vi "Worker List UI.vi"(11 "Opened from Block":bool) -> (3 "Selected Worker Lib":path)   [LabVIEW 2022 SP3, in "FlexBlocks Support.lvlib"]
uses:
  FlexBlocks Support.lvlib
  <vilib>/IlluminatedG/IG AutoComplete/AutoComplete/AutoComplete.lvlib
panel:
  out "Prompt":string
  in  "Select Worker":bool
  in  "Refresh Workers":bool
  in  "Refresh Worker":bool
  out "Icon":picture
  in  "New Variant":bool
  in  "Enable Variants":bool
  in  "Open Worker":bool
  in  "Values":string(tree)
  in  "New Worker":bool
  in  "Variant":i32(listbox)
  in  "Worker Search":string
  in  "Clear Search":bool
  out "Worker Name":string
  in  "Workers":i32(listbox)
  # "No variants for the selected worker"
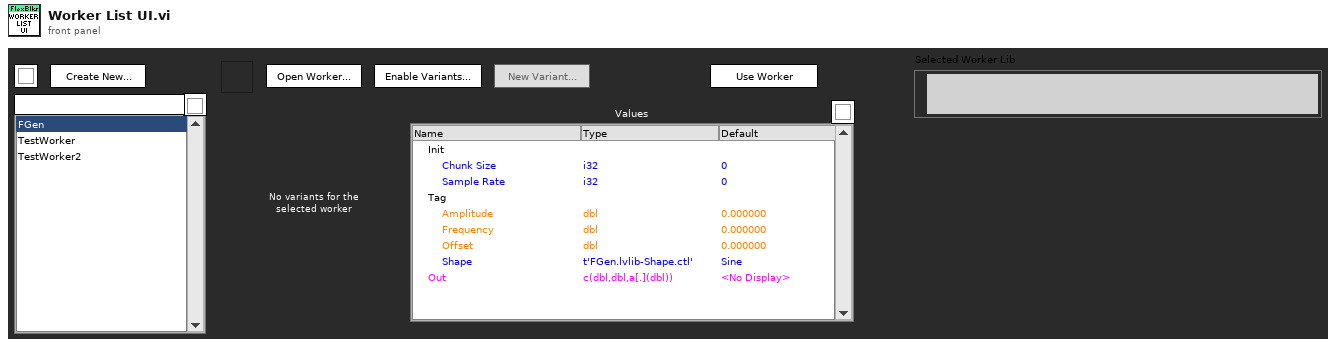
[diagram p1: front panel]
types:
  T1 = typedef "FlexBlocks Support.lvlib/UI State.ctl" = enum16{"Init", "Load", "Ready", "Run", "Cleanup", "Close"}
  T2 = enum8{"Enabled", "Disabled", "Disabled and Grayed Out"}
  T3 = enum32{"Invalid", "Standard", "Closed", "Hidden", "Minimized", "Maximized"}
  T4 = typedef "FlexBlocks Support.lvlib/Action Selections.ctl" = cluster{"Init":bool, "Start":bool, "Run":bool, "Stop":bool, "Close":bool}
  T5 = typedef "FlexBlocks Support.lvlib/Worker Info.ctl" = cluster{"Name":string, "Icon":T6, "Index":i32, "Variants":map{string, T7}}
  T6 = typedef "imagedata.ctl" = cluster{"image type":i32, "image depth":i32, "image":u8[], "mask":u8[], "colors":u32[], "Rectangle":cluster{"left":i16, "top":i16, "right":i16, "bottom":i16}}
  T7 = typedef "FlexBlocks Support.lvlib/Worker Variant.ctl" = cluster{"Name":string, "Icon":T6}
  T8 = typedef "FlexBlocks Support.lvlib/Type Descriptor.ctl" = cluster{"Name":string, "Direction":T9, "Default":variant, "Min":variant, "Max":variant, "Step":variant, "Value Mode":T10, "Color":u32, "Options":string[], "Type String":string, "Item Path":path, "Required":bool, "Connpane Index":i32, "Special Terminal":T11, "Sort":i32}
  T9 = typedef "FlexBlocks Support.lvlib/Terminal Direction.ctl" = enum16{"Sink", "Source"}
  T10 = typedef "FlexBlocks Support.lvlib/Value Mode.ctl" = enum16{"Normal", "Range", "Select"}
  T11 = typedef "FlexBlocks Support.lvlib/Special Terminal.ctl" = enum16{"None", "Action", "Init", "Tag", "State in", "State out", "Error"}
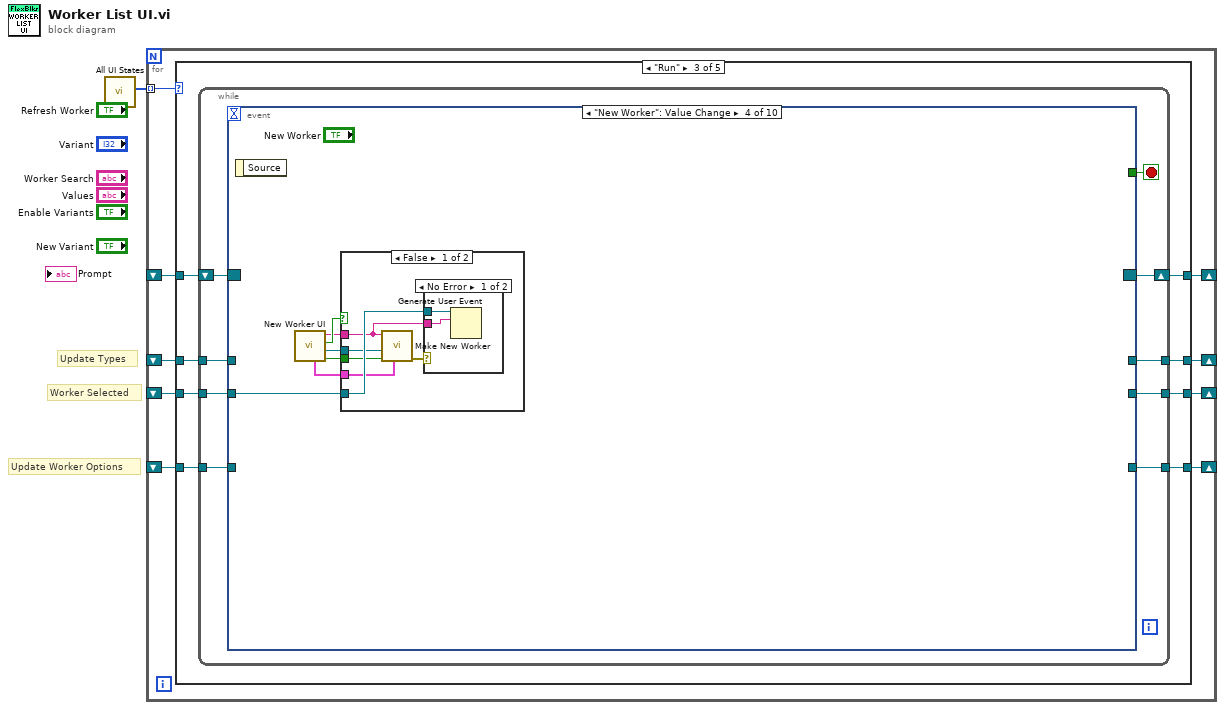
[diagram p0: block diagram]
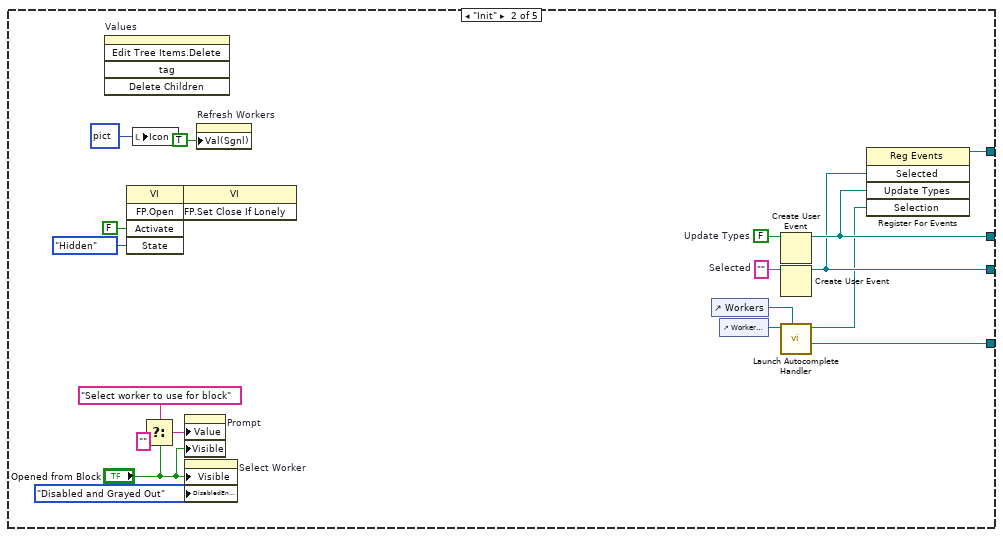
[diagram p3: hidden frame]
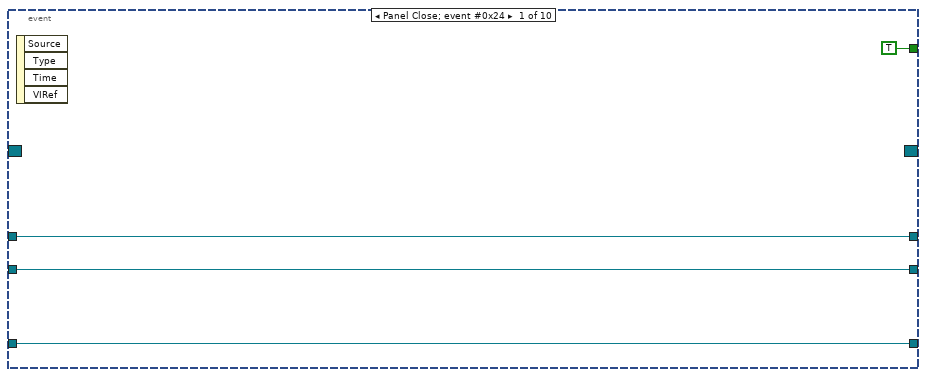
[diagram p4: hidden frame]
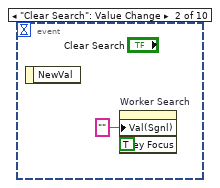
[diagram p5: hidden frame]
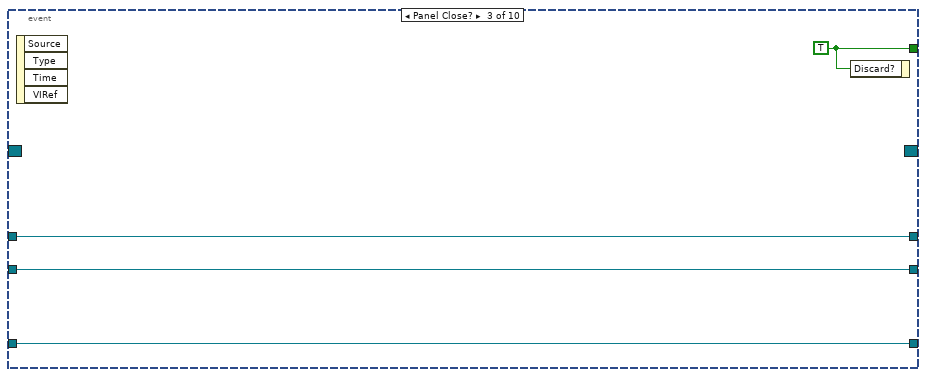
[diagram p6: hidden frame]
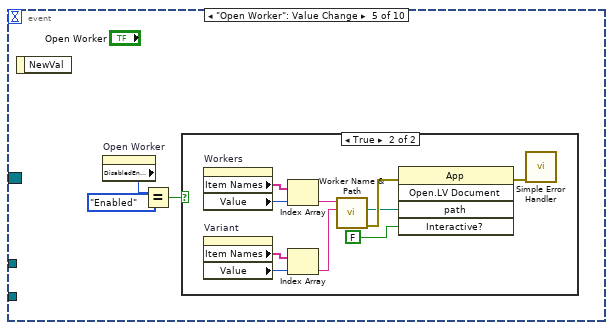
[diagram p9: hidden frame]
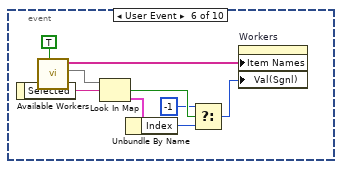
[diagram p11: hidden frame]
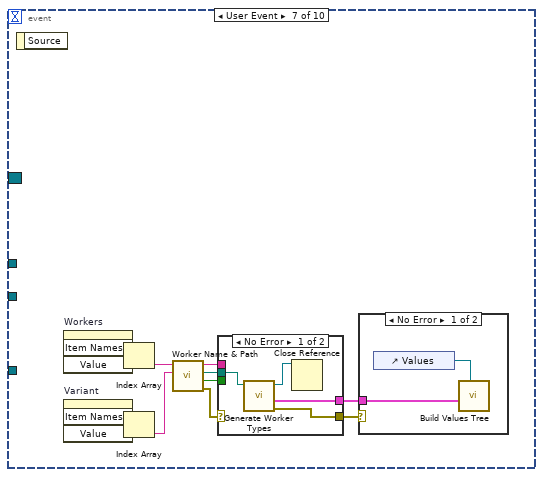
[diagram p12: hidden frame]
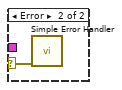
[diagram p13: hidden frame]
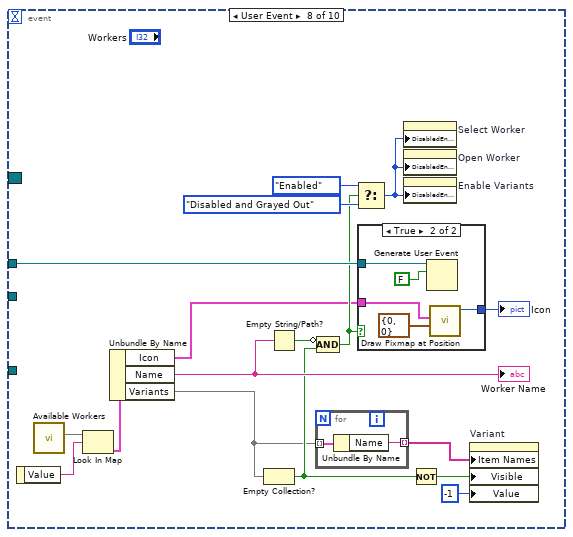
[diagram p15: hidden frame]
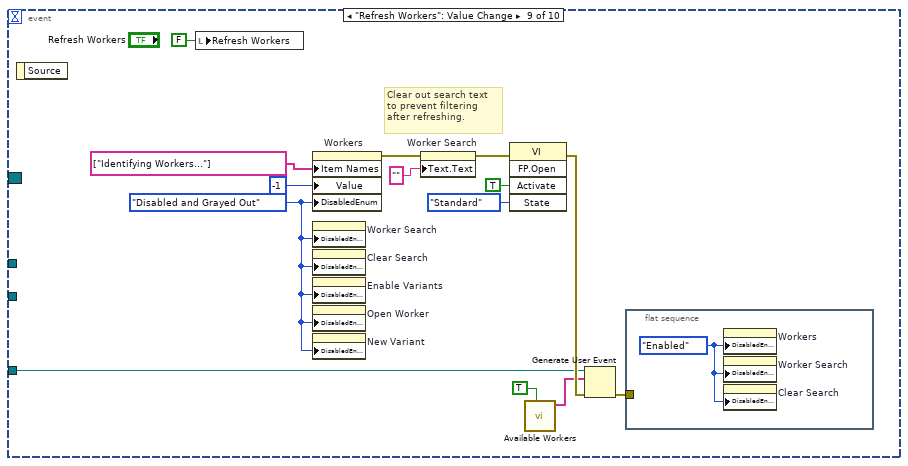
[diagram p17: hidden frame]
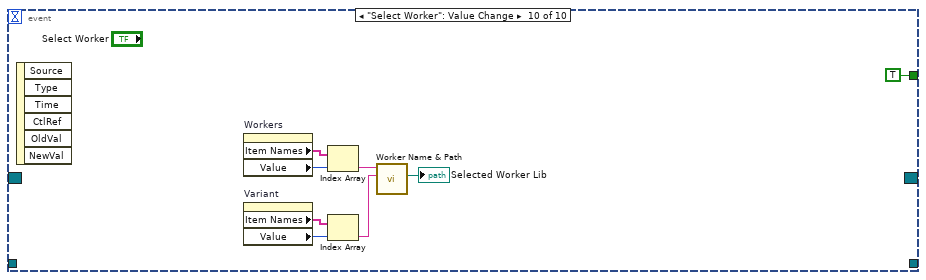
[diagram p18: hidden frame]
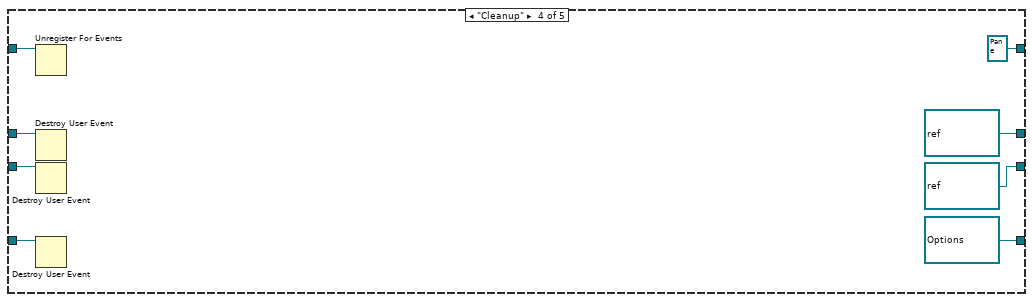
[diagram p19: hidden frame]
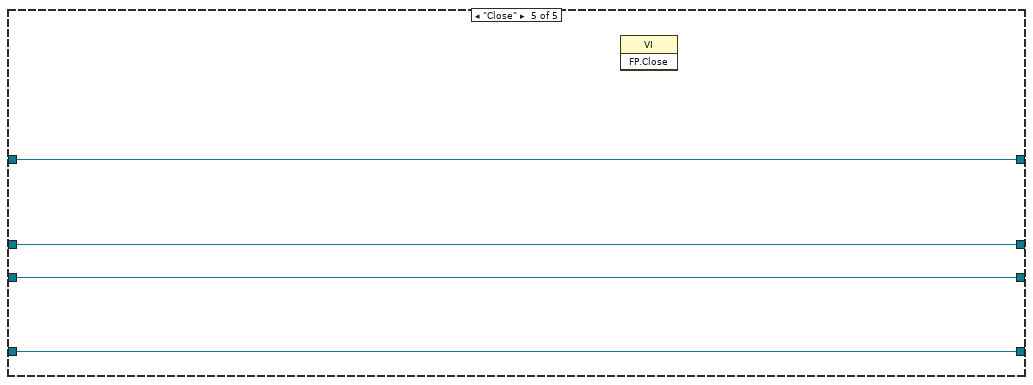
[diagram p20: hidden frame]
diagram:
  # "Update Worker Options"
  # "Worker Selected"
  # "Update Types"
  n1 = call "All UI States.vi"() -> ("All UI States"=w1:T1[])  [unwired: 11 in]
  n2 = for {
    tunnel: w1 -> [w10] mode=indexing
    shift-right: [w9] -> _
    shift-left: _ -> [w6]
    shift-right: [w8] -> _
    shift-left: _ -> [w5]
    shift-right: [w7] -> _
    shift-left: _ -> [w4]
    shift-right: [w3] -> _
    shift-left: _ -> [w2]
    n3 = case shown="\"Run\"" w10 {
      tunnel: [w14 w23 w41 refnum<event-registration> refnum ("Event Registration Refnum") w176] -> w9
      tunnel: [w13 w29 w38 refnum<user-event> refnum ("Update Types") w175] -> w8
      tunnel: [w12 w28 w37 refnum<user-event> refnum ("Selected") w174] -> w7
      tunnel: w6 -> [w14 _ w42 w172 w176]
      tunnel: w5 -> [w13 _ w40 w171 w175]
      tunnel: w4 -> [w12 _ w39 w170 w174]
      tunnel: [w11 w25 w35 refnum<user-event> refnum ("New Options Event") w173] -> w3
      tunnel: w2 -> [w11 _ w36 w167 w173]
      frame Default {
      }
      frame "Init" {
        w30 = FALSE  # Update Types
        w31 = ""  # Selected
        n4 = invoke on="Values" class="Tree (strict)" method="Edit Tree Items.Delete"() -> ()  [unwired: 5 in, 5 out]
        n5 = invoke class="VI" method="FP.Open"("Activate"=FALSE ("Activate?"), "State"=T3."Hidden") -> (reference out=w20:refnum<vi>, error out=w21:errorcluster)  [unwired: 3 in, 3 out]
        n6 = local write "Icon"(picture data[5B] ("empty picture")) -> ()
        n7 = Select(t="Select worker to use for block" ("Prompt"), s="Opened from Block", f="") -> (s? t:f=w17:string)
        n8 = invoke class="VI" method="FP.Set Close If Lonely"(reference=w20, error in=w21) -> ()  [unwired: 1 in, 3 out]
        n9 = property on="Prompt" class="Str"("Value"=w17, "Visible"="Opened from Block") -> ()  [unwired: 2 in, 2 out]
        n10 = property on="Select Worker" class="Bool"("Visible"="Opened from Block", "DisabledEnum"=T2."Disabled and Grayed Out" ("Disabled")) -> ()  [unwired: 2 in, 2 out]
        n11 = property on="Refresh Workers" class="Bool (strict)"("Val(Sgnl)"=TRUE ("Value (Signaling)")) -> ()  [unwired: 2 in, 2 out]
        n12 = control-ref of="Workers"() -> (w26:refnum<vi>)
        n13 = control-ref of="Worker Search"() -> (w27:refnum<vi>)
        n14 = Create User Event(user event datatype=w30) -> (user event=w29:refnum<user-event>)  [unwired: 1 in, 1 out]
        n15 = Create User Event(user event datatype=w31) -> (user event=w28:refnum<user-event>)  [unwired: 1 in, 1 out]
        n16 = call <vilib>:"Launch Autocomplete Handler.vi"("ListBox Refnum (Popup)"=w26, "Str Refnum"=w27) -> ("New Options Event"=w25:refnum<user-event>, "Selection"=w22:refnum<user-event>)  [unwired: 6 in, 2 out]
        n17 = register-events(w28, w29, w22) -> (reference out=w23:refnum<event-registration>)  [unwired: 2 in, 1 out]
      }
      frame "Run" {
        n18 = while {
          shift-right: [w44] -> w41
          shift-left: w42 -> [w45]
          tunnel: w40 -> [w50]
          tunnel: w39 -> [w49]
          tunnel: [w48] -> w38
          tunnel: [w47] -> w37
          tunnel: w36 -> [w46]
          tunnel: [w43] -> w35
          stop <- w51 stop-if-true
          n19 = event shown="[3] \"New Worker\": Value Change" {
            selector: w45 -> [_ _ _ _ _ _ _ _ _ _]
            dyn-events: [_ _ _ _ _ _ _ _ _ _] -> w44
            timeout: _ -> [_ _ _ _ _ _ _ _ _ _]
            tunnel: [TRUE ("Discard?") _ w61 _ _ _ _ _ _ TRUE ("Discard?")] -> w51
            tunnel: w50 -> [w54 _ w60 _ _ _ _ w131 _ _]
            tunnel: w49 -> [w53 _ w59 w63 _ _ _ _ _ _]
            tunnel: [w54 _ w60 _ _ _ _ _ _ _] -> w48
            tunnel: [w53 _ w59 _ _ _ _ _ _ _] -> w47
            tunnel: w46 -> [w52 _ w58 _ _ _ _ _ w147 _]
            tunnel: [w52 _ w58 _ _ _ _ _ _ _] -> w43
            event Panel Close; event #0x24 {
              n20 = event-data() -> ()  [unwired: 1 in, 4 out]
            }
            event "Clear Search": Value Change {
              n21 = event-data() -> ()  [unwired: 1 in, 1 out]
              n22 = property on="Worker Search" class="Str"("Val(Sgnl)"="" ("Value (Signaling)"), "Key Focus"=TRUE) -> ()  [unwired: 2 in, 2 out]
            }
            event Panel Close? {
              w61 = TRUE ("Discard?")
              n23 = event-data() -> ()  [unwired: 1 in, 4 out]
              n24 = event-data("Discard?"=w61) -> ()  [unwired: 1 in, 1 out]
            }
            event "New Worker": Value Change {
              n25 = event-data() -> ()  [unwired: 1 in, 1 out]
              n26 = call "New Worker UI.vi"() -> ("New Project?"=w64:bool, "Project"=w65:refnum<vi>, "Cancelled?"=w67:bool, "New Name"=w66:string, "Selected Actions"=w62:T4)  [unwired: 7 in]
              n27 = case shown="False" w67 {
                tunnel: w66 -> [w72 _]
                tunnel: w65 -> [w71 _]
                tunnel: w64 -> [w70 _]
                tunnel: w63 -> [w73 _]
                tunnel: w62 -> [w68 _]
                frame False {
                  n28 = call "Make New Worker.vi"("Selected Actions"=w68, "New Project?"=w70, "Add to Project (None)"=w71, "New Worker Name"=w72) -> ("error out"=w69:errorcluster)  [unwired: 7 in]
                  n29 = case shown="No Error" w69 {
                    tunnel: w73 -> [w75 _]
                    tunnel: w72 -> [w74 _]
                    frame No Error {
                      n30 = Generate User Event(user event=w75, event data cluster=w74) -> ()  [unwired: 2 in, 2 out]
                    }
                    frame Error {
                    }
                  }
                }
                frame True {
                }
              }
            }
            event "Open Worker": Value Change {
              n31 = event-data() -> ()  [unwired: 1 in, 1 out]
              n32 = property on="Open Worker" class="Bool"() -> ("DisabledEnum"=w78:T2)  [unwired: 2 in, 2 out]
              n33 = Equal?(x=w78, y=T2."Enabled") -> (x = y?=w76:bool)
              n34 = case shown="True" w76 {
                frame False {
                }
                frame True {
                  n35 = property on="Workers" class="LstBox (strict)"() -> ("Item Names"=w87:string[], "Value"=w86:i32)  [unwired: 2 in, 2 out]
                  n36 = property on="Variant" class="LstBox (strict)"() -> ("Item Names"=w84:string[], "Value"=w85:i32)  [unwired: 2 in, 2 out]
                  n37 = Index Array(array=w87, index=w86) -> (element=w83:string)
                  n38 = Index Array(array=w84, index=w85) -> (element=w82:string)
                  n39 = call "Worker Name & Path.vi"("Variant"=w82, "Worker"=w83) -> ("error out"=w88:errorcluster, "lvlib Path"=w81:path)  [unwired: 5 in, 3 out]
                  n40 = invoke class="App" method="Open.LV Document"(error in=w88, "path"=w81, "Interactive?"=FALSE) -> (error out=w79:errorcluster)  [unwired: 2 in, 4 out]
                  n41 = call <vilib>:"Simple Error Handler.vi"("error in (no error)"=w79) -> ()  [unwired: 4 in, 5 out]
                }
              }
            }
            event User Event {
              n42 = event-data() -> ("Selected"=w95:string)  [unwired: 1 in]
              n43 = call "Available Workers.vi"("Refresh? (F)"=TRUE) -> ("Workers Map"=w96:map{string, T5}, "Names"=w89:string[])  [unwired: 9 in]
              n44 = Look In Map(map=w96, key=w95) -> (key not found?=w92:bool, value=w94:T5)  [unwired: 1 in]
              n45 = Unbundle By Name(w94) -> ("Index"=w93:i32)
              n46 = Select(t=-1, s=w92, f=w93) -> (s? t:f=w90:i32)
              n47 = property on="Workers" class="LstBox (strict)"("Item Names"=w89, "Val(Sgnl)"=w90) -> ()  [unwired: 2 in, 2 out]
            }
            event User Event {
              n48 = event-data() -> ()  [unwired: 1 in, 1 out]
              n49 = property on="Workers" class="LstBox (strict)"() -> ("Item Names"=w109:string[], "Value"=w108:i32)  [unwired: 2 in, 2 out]
              n50 = property on="Variant" class="LstBox (strict)"() -> ("Item Names"=w106:string[], "Value"=w107:i32)  [unwired: 2 in, 2 out]
              n51 = Index Array(array=w109, index=w108) -> (element=w105:string)
              n52 = Index Array(array=w106, index=w107) -> (element=w104:string)
              n53 = call "Worker Name & Path.vi"("Variant"=w104, "Worker"=w105) -> ("error out"=w103:errorcluster, "Is Worker Variant"=w102:bool, "lvlib Path"=w101:path, "Display Name"=w100:string)  [unwired: 5 in, 1 out]
              n54 = case shown="No Error" w103 {
                selector: w103 -> [_ w117]
                tunnel: w102 -> [_ _]
                tunnel: w101 -> [w115 _]
                tunnel: w100 -> [_ _]
                tunnel: [w116 w117] -> w99
                tunnel: [w114 _] -> w98
                frame No Error {
                  n55 = call "Generate Worker Types.vi"("Worker lvlib"=w115) -> ("error out"=w116:errorcluster, "Types"=w114:T8[], "Worker VI"=w113:refnum<vi>)  [unwired: 7 in, 1 out]
                  n56 = Close Reference(reference=w113) -> ()  [unwired: 1 in, 1 out]
                }
                frame Error {
                }
              }
              n57 = case shown="No Error" w99 {
                selector: w99 -> [_ w112]
                tunnel: w98 -> [w111 _]
                frame No Error {
                  n58 = control-ref of="Values"() -> (w110:refnum<vi>)
                  n59 = call "Build Values Tree.vi"("Tree"=w110, "Types"=w111) -> ()  [unwired: 10 in]
                }
                frame Error {
                  n60 = call <vilib>:"Simple Error Handler.vi"("error in (no error)"=w112) -> ()  [unwired: 4 in, 5 out]
                }
              }
            }
            event User Event {
              n61 = event-data() -> ("Value"=w134:string)  [unwired: 1 in]
              n62 = call "Available Workers.vi"() -> ("Workers Map"=w119:map{string, T5})  [unwired: 10 in, 1 out]
              n63 = Look In Map(map=w119, key=w134) -> (value=w118:T5)  [unwired: 1 in, 1 out]
              n64 = Unbundle By Name(w118) -> ("Icon"=w125:T6, "Name"=w130:string, "Variants"=w120:map{string, T7})
              "Worker Name" <- w130
              n65 = Empty Collection?(1:w120) -> (0:w121:bool)
              n66 = Empty String/Path?(string/path=w130) -> (empty?=w129:bool)
              n67 = for {
                tunnel: w120 -> [w136] mode=indexing
                tunnel: [w135] -> w123 mode=indexing
                n68 = Unbundle By Name(w136) -> ("Name"=w135:string)
              }
              n69 = Compound Arithmetic op=AND(invert w129, w121) -> (w126:bool)
              n70 = Select(t=T2."Enabled" ("Disabled"), s=w126, f=T2."Disabled and Grayed Out" ("Disabled")) -> (s? t:f=w122:T2)
              n71 = case shown="True" w126 {
                tunnel: w131 -> [_ w141]
                tunnel: w125 -> [_ w138]
                tunnel: [_ w137] -> w124
                frame False {
                }
                frame True {
                  n72 = Generate User Event(user event=w141, event data cluster=FALSE ("event data")) -> ()  [unwired: 2 in, 2 out]
                  n73 = call "Draw Pixmap at Position.vi"("Position"=cluster{"left":i16, "top":i16} {"left"=0, "top"=0}, "Pixmap"=w138) -> ("2D Picture"=w137:picture)  [unwired: 9 in]
                }
              }
              "Icon" <- w124
              n74 = property on="Select Worker" class="Bool"("DisabledEnum"=w122) -> ()  [unwired: 2 in, 2 out]
              n75 = property on="Open Worker" class="Bool"("DisabledEnum"=w122) -> ()  [unwired: 2 in, 2 out]
              n76 = property on="Enable Variants" class="Bool"("DisabledEnum"=w122) -> ()  [unwired: 2 in, 2 out]
              n77 = Not(x=w121) -> (.not. x?=w133:bool)
              n78 = property on="Variant" class="LstBox (strict)"("Item Names"=w123, "Visible"=w133, "Value"=-1 ("Variant")) -> ()  [unwired: 2 in, 2 out]
            }
            event "Refresh Workers": Value Change {
              w151 = T2."Disabled and Grayed Out" ("Disabled")
              # "Clear out search text to prevent filtering after refreshing."
              n79 = event-data() -> ()  [unwired: 1 in, 1 out]
              n80 = local write "Refresh Workers"(FALSE ("Refresh Workers")) -> ()
              n81 = property on="Workers" class="LstBox (strict)"("Item Names"=string[] ["Identifying Workers..."], "Value"=-1 ("Workers"), "DisabledEnum"=w151) -> (error out=w144:errorcluster)  [unwired: 2 in, 1 out]
              n82 = property on="Worker Search" class="Str"("DisabledEnum"=w151) -> ()  [unwired: 2 in, 2 out]
              n83 = property on="Clear Search" class="Bool"("DisabledEnum"=w151) -> ()  [unwired: 2 in, 2 out]
              n84 = property on="Enable Variants" class="Bool"("DisabledEnum"=w151) -> ()  [unwired: 2 in, 2 out]
              n85 = property on="Open Worker" class="Bool"("DisabledEnum"=w151) -> ()  [unwired: 2 in, 2 out]
              n86 = property on="New Variant" class="Bool"("DisabledEnum"=w151) -> ()  [unwired: 2 in, 2 out]
              n87 = property on="Worker Search" class="Str"(error in=w144, "Text.Text"="") -> (error out=w142:errorcluster)  [unwired: 1 in, 1 out]
              n88 = invoke class="VI" method="FP.Open"(error in=w142, "Activate"=TRUE ("Activate?"), "State"=T3."Standard") -> (error out=w155:errorcluster)  [unwired: 2 in, 4 out]
              n89 = call "Available Workers.vi"("Refresh? (F)"=TRUE) -> ("Names"=w145:string[])  [unwired: 9 in, 1 out]
              n90 = Generate User Event(user event=w147, event data cluster=w145, error in=w155) -> (error out=w146:errorcluster)  [unwired: 1 in, 1 out]
              n91 = flat-sequence {
                tunnel: w146 -> [_]
                frame #0 {
                  w156 = T2."Enabled" ("Disabled")
                  n92 = property on="Workers" class="LstBox (strict)"("DisabledEnum"=w156) -> ()  [unwired: 2 in, 2 out]
                  n93 = property on="Worker Search" class="Str"("DisabledEnum"=w156) -> ()  [unwired: 2 in, 2 out]
                  n94 = property on="Clear Search" class="Bool"("DisabledEnum"=w156) -> ()  [unwired: 2 in, 2 out]
                }
              }
            }
            event "Select Worker": Value Change {
              n95 = event-data() -> ()  [unwired: 1 in, 6 out]
              n96 = property on="Workers" class="LstBox (strict)"() -> ("Item Names"=w164:string[], "Value"=w163:i32)  [unwired: 2 in, 2 out]
              n97 = property on="Variant" class="LstBox (strict)"() -> ("Item Names"=w161:string[], "Value"=w162:i32)  [unwired: 2 in, 2 out]
              n98 = Index Array(array=w164, index=w163) -> (element=w160:string)
              n99 = Index Array(array=w161, index=w162) -> (element=w159:string)
              n100 = call "Worker Name & Path.vi"("Variant"=w159, "Worker"=w160) -> ("lvlib Path"=→"Selected Worker Lib":path)  [unwired: 5 in, 4 out]
            }
          }
        }
      }
      frame "Cleanup" {
        n101 = Unregister For Events(event registration refnum=w172) -> ()  [unwired: 1 in, 1 out]
        n102 = Destroy User Event(user event=w171) -> ()  [unwired: 1 in, 1 out]
        n103 = Destroy User Event(user event=w170) -> ()  [unwired: 1 in, 1 out]
        n104 = Destroy User Event(user event=w167) -> ()  [unwired: 1 in, 1 out]
      }
      frame "Close" {
        n105 = invoke class="VI" method="FP.Close"() -> ()  [unwired: 3 in, 3 out]
      }
    }
  }
